vi "QVA_DataProbe.vi"(11 "QueueOut":refnum<queue>) -> (2 "Value String":string, 3 "Boolean":bool)   [LabVIEW 2016]
doc: "Probe für Single Element Queue Variant Attributes\n\n18.12.13 / sige"
uses:
  private/QVA.VariableDataTypeDef.ctl
panel:
  in  "Multicolumn Listbox":i32(listbox)
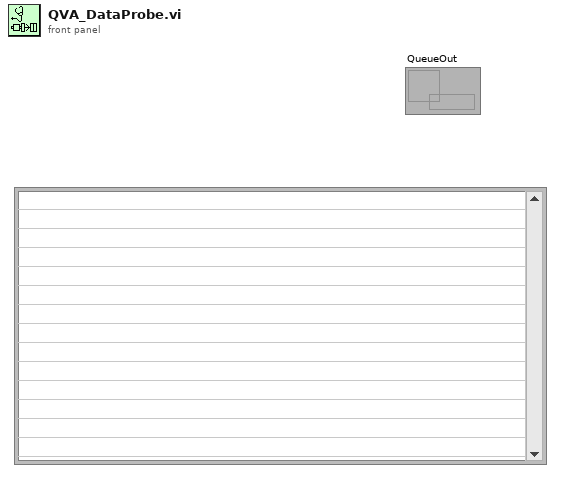
[diagram p1: front panel]
types:
  T1 = typedef "QVA.VariableDataTypeDef.ctl" = cluster{"Type":string, "Data":variant}
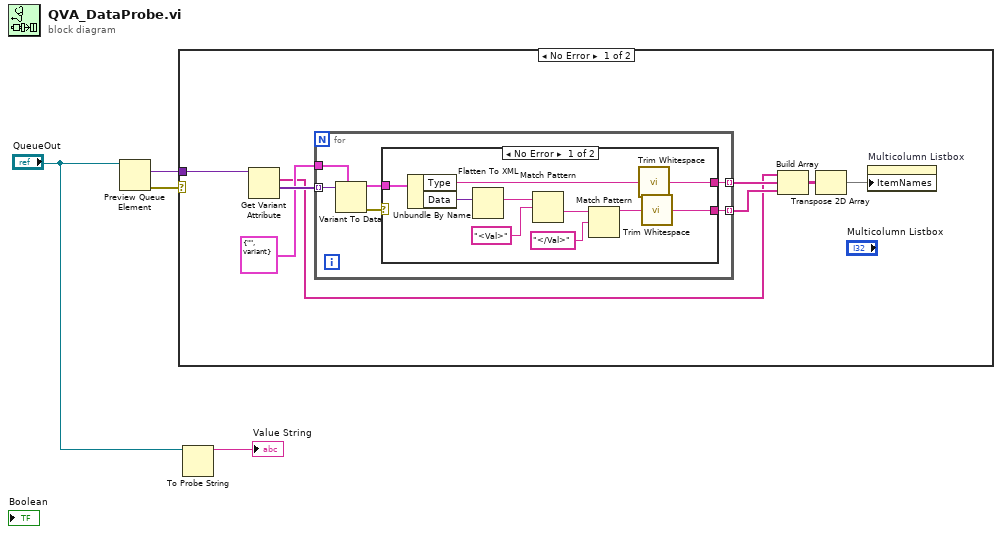
[diagram p0: block diagram]
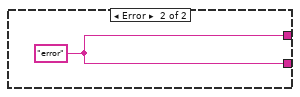
[diagram p2: hidden frame]
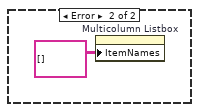
[diagram p3: hidden frame]
diagram:
  n1 = Preview Queue Element(queue="QueueOut") -> (element=w2:variant, error out=w1:errorcluster)  [unwired: 2 in, 2 out]
  n2 = case shown="No Error" w1 {
    tunnel: w2 -> [w12 _]
    frame No Error {
      n3 = Get Variant Attribute(Variant=w12) -> (names=w7:string[], values=w11:variant[])  [unwired: 3 in, 2 out]
      n4 = for {
        tunnel: w11 -> [w18] mode=indexing
        tunnel: T1 {"Type"="", "Data"=variant} -> [w17]
        tunnel: [w14] -> w9 mode=indexing
        tunnel: [w13] -> w8 mode=indexing
        n5 = Variant To Data(type=w17, Variant=w18) -> (data=w15:T1, error out=w16:errorcluster)  [unwired: 1 in]
        n6 = case shown="No Error" w16 {
          tunnel: w15 -> [w28 _]
          tunnel: [w19 w29] -> w14
          tunnel: [w20 w29] -> w13
          frame No Error {
            n7 = Unbundle By Name(w28) -> ("Type"=w27:string, "Data"=w23:variant)
            n8 = Flatten To XML(anything=w23) -> (xml string=w24:string)
            n9 = Match Pattern(string=w24, regular expression="<Val>") -> (after substring=w25:string)  [unwired: 1 in, 3 out]
            n10 = Match Pattern(string=w25, regular expression="</Val>") -> (before substring=w22:string)  [unwired: 1 in, 3 out]
            n11 = call <vilib>:"Trim Whitespace.vi"("string"=w27) -> ("trimmed string"=w19:string)  [unwired: 1 in]
            n12 = call <vilib>:"Trim Whitespace.vi"("string"=w22) -> ("trimmed string"=w20:string)  [unwired: 1 in]
          }
          frame Error {
            w29 = "error"
          }
        }
      }
      n13 = Build Array(w7, w9, w8) -> (w6:string[][])
      n14 = Transpose 2D Array(2D array=w6) -> (transposed array=w5:string[][])
      n15 = property on="Multicolumn Listbox" class="MCListbox (strict)"("ItemNames"=w5) -> ()  [unwired: 2 in, 2 out]
    }
    frame Error {
      n16 = property on="Multicolumn Listbox" class="MCListbox (strict)"("ItemNames"=string[][] [] ("Item Names")) -> ()  [unwired: 2 in, 2 out]
    }
  }
  n17 = To Probe String(7:"QueueOut") -> (3:→"Value String":string)  [unwired: 2 in, 1 out]
